vi "ni579x Configure Mixer.vi"(0 "Register Bus":T1, 1 "scope":string(combo)="rx", 5 "frequency [Hz]":dbl format="%#_6p", 9 "LO source":string(combo)="LO1", 11 "Error In":errorcluster) -> (4 "Register Bus (out)":T1, 6 "coerced frequency [Hz]":dbl format="%#_6p", 15 "Error Out":errorcluster)   [LabVIEW 2015, in "ni579x Config v2 Host.lvlib"]
doc: "Configures the mixer (RF up/down-coverter) by enabling the LO, setting the LO frequency, configuring the LO filter, and making any necessary routes.\n\n<B>Input Parameters</B>\n\n<B>Register Bus</B> The Register Bus object created by the ni579x Open VI and used as the session handle for the NI-579x Configuration Design Library.\n\n<B>scope</B> Specifies which mixer to configure. Can be \"rx\" or \"tx\".\n\n<B>frequency [Hz]</B> Specifies the frequency to tune the LO or the frequency of the incoming LO (if using an external LO source)\n\n<B>LO source</B> The source of the local oscillator used by the specified mixer. \"LO1\" for the internal LO. \"LO In\" to use an external LO source.\n\n<B>Output Parameters</B>\n\n<B>Register Bus (out)</B> The Register Bus object created by the ni579x Open VI and used as the session handle for the NI-579x Configuration Design Library.\n\n<B>coerced frequency [Hz]</B> The actual frequency the LO was tuned to."
uses:
  <instrlib>/ni579x/Config/v2/Host/ni579x Config v2 Host.lvlib
  <instrlib>/_niInstr/Register Bus/v0/Host/Public/Register Bus Session.ctl
  <instrlib>/_niInstr/Register Bus/v0/Host/Private/Session Data.ctl
  <instrlib>/_niInstr/Register Bus/v0/Host/niInstr Register Bus v0 Host.lvlib
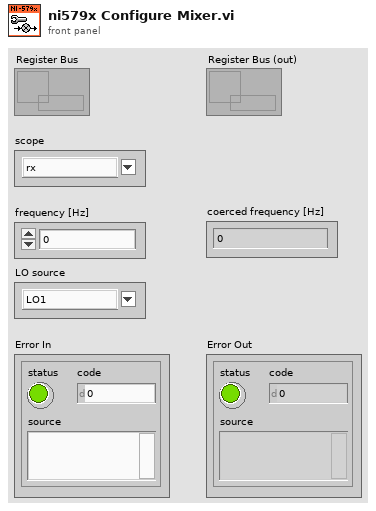
[diagram p1: front panel]
types:
  T1 = typedef "niInstr Register Bus v0 Host.lvlib/Register Bus Session.ctl" = refnum<queue>
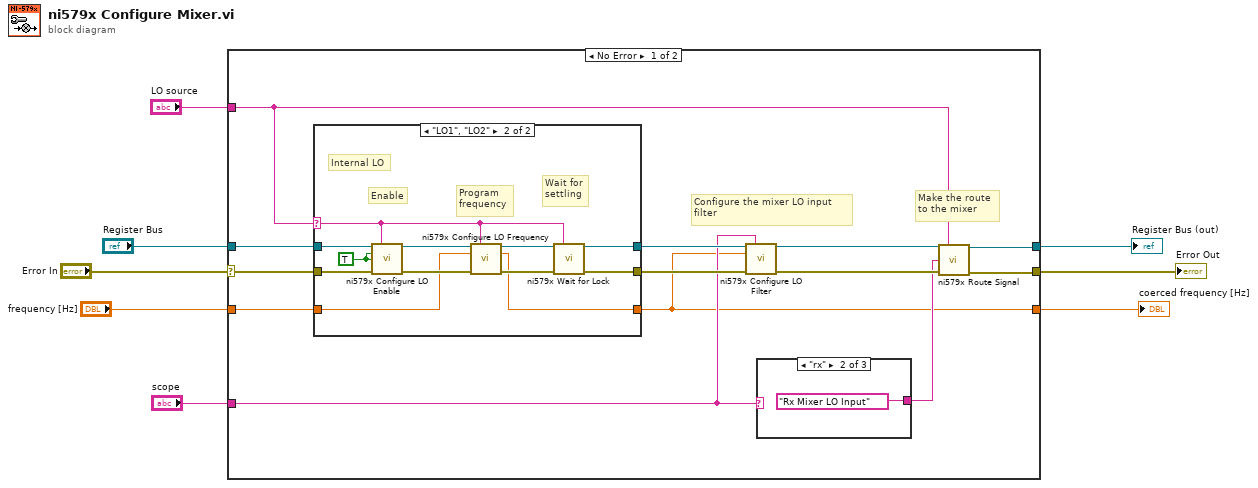
[diagram p0: block diagram]
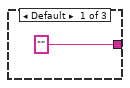
[diagram p2: hidden frame]
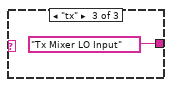
[diagram p3: hidden frame]
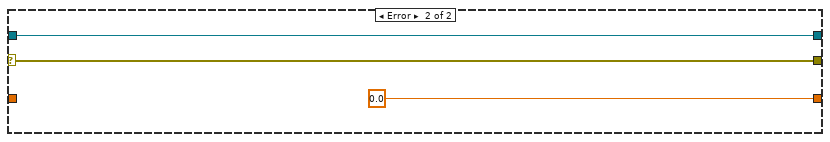
[diagram p5: hidden frame]
diagram:
  n1 = case shown="No Error" "Error In" {
    selector: "Error In" -> [w20 w42]
    tunnel: [w9 w42] -> w7
    tunnel: "Register Bus" -> [w21 w41]
    tunnel: "frequency [Hz]" -> [w19 _]
    tunnel: [w15 w41] -> w4
    tunnel: [w10 0.0 ("coerced attenuation [dB]")] -> w3
    tunnel: "scope" -> [w12 _]
    tunnel: "LO source" -> [w14 _]
    frame No Error {
      # "Make the route\nto the mixer"
      # "Configure the mixer LO input \nfilter"
      n2 = case shown="\"LO1\", \"LO2\"" w14 {
        selector: w14 -> [_ w31]
        tunnel: w21 -> [w27 w39]
        tunnel: w20 -> [w26 w38]
        tunnel: [w27 w30] -> w18
        tunnel: [w26 w29] -> w17
        tunnel: w19 -> [w25 w34]
        tunnel: [w25 w28] -> w10
        frame Default {
          # "External LO"
        }
        frame "LO1", "LO2" {
          w37 = TRUE ("enable?")
          # "Wait for\nsettling"
          # "Program\nfrequency"
          # "Enable"
          # "Internal LO"
          n3 = call <instrlib>:"ni579x Configure LO Enable.vi"("Register Bus"=w39, "scope"=w31, "enable?"=w37, "wait for enable completion?"=w37, "Error In"=w38) -> ("Register Bus (out)"=w36:T1, "Error Out"=w35:errorcluster)  [unwired: 9 in]
          n4 = call <instrlib>:"ni579x Configure LO Frequency.vi"("Register Bus"=w36, "scope"=w31, "frequency [Hz]"=w34, "Error In"=w35) -> ("Register Bus (out)"=w33:T1, "coerced frequency [Hz]"=w28:dbl, "Error Out"=w32:errorcluster)  [unwired: 9 in]
          n5 = call <instrlib>:"ni579x Wait for Lock.vi"("Register Bus"=w33, "scope"=w31, "Error In"=w32) -> ("Register Bus (out)"=w30:T1, "Error Out"=w29:errorcluster)  [unwired: 11 in]
        }
      }
      n6 = call <instrlib>:"ni579x Configure LO Filter.vi"("Register Bus"=w18, "scope"=w12, "frequency [Hz]"=w10, "Error In"=w17) -> ("Register Bus (out)"=w16:T1, "Error Out"=w13:errorcluster)  [unwired: 9 in, 1 out]
      n7 = case shown="\"rx\"" w12 {
        tunnel: ["" ("destination") "Rx Mixer LO Input" ("destination") "Tx Mixer LO Input" ("destination")] -> w11
        frame Default {
        }
        frame "rx" {
        }
        frame "tx" {
        }
      }
      n8 = call <instrlib>:"ni579x Route Signal.vi"("Register Bus"=w16, "source"=w14, "destination"=w11, "Error In"=w13) -> ("Register Bus (out)"=w15:T1, "Error Out"=w9:errorcluster)  [unwired: 10 in]
    }
    frame Error {
    }
  }
  "Register Bus (out)" <- w4
  "Error Out" <- w7
  "coerced frequency [Hz]" <- w3
